vi "SubVI-Config-AI.vi"(8 "error in (no error)":errorcluster, 10 "Channels":T1(array[cluster])=[{" Physical Channel"="Dev2/ai0", "Name"="V_R", "Vmax"=10.0, "Vmin"=-10.0}, {" Physical Channel"="Dev2/ai1", "Name"="V_C", "Vmax"=10.0, "Vmin"=-10.0}, {" Physical Channel"="Dev2/ai2", "Name"="V_S", "Vmax"=10.0, "Vmin"=-10.0}], 11 "Timing Params":T2={"Trigger Level"=0.0, "Sample Rate"=0.0, "N Samples"=0, "Trigger Slope"=10280, "Enable"=FALSE} {"Trigger Slope" items=["Rising"=10171, "Falling"=10280]}) -> (0 "error out":errorcluster, 3 "Refnum out":refnum<k21>)   [LabVIEW 2023]
uses:
  <vilib>/DAQmx/create/channels.llb/DAQmx Create Channel (AI-Voltage-Basic).vi
  <vilib>/DAQmx/configure/timing.llb/DAQmx Timing (Sample Clock).vi
  <vilib>/DAQmx/configure/trigger.llb/DAQmx Start Trigger (Analog Edge).vi
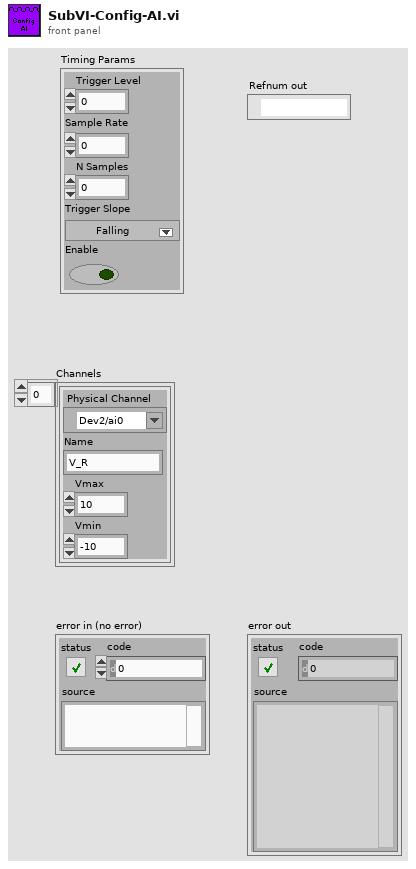
[diagram p1: front panel]
types:
  T1 = cluster{" Physical Channel":tag, "Name":string, "Vmax":dbl, "Vmin":dbl}[]
  T2 = cluster{"Trigger Level":dbl, "Sample Rate":dbl, "N Samples":i32, "Trigger Slope":i32, "Enable":bool}
  T3 = cluster{" Physical Channel":tag, "Name":string, "Vmax":dbl, "Vmin":dbl}
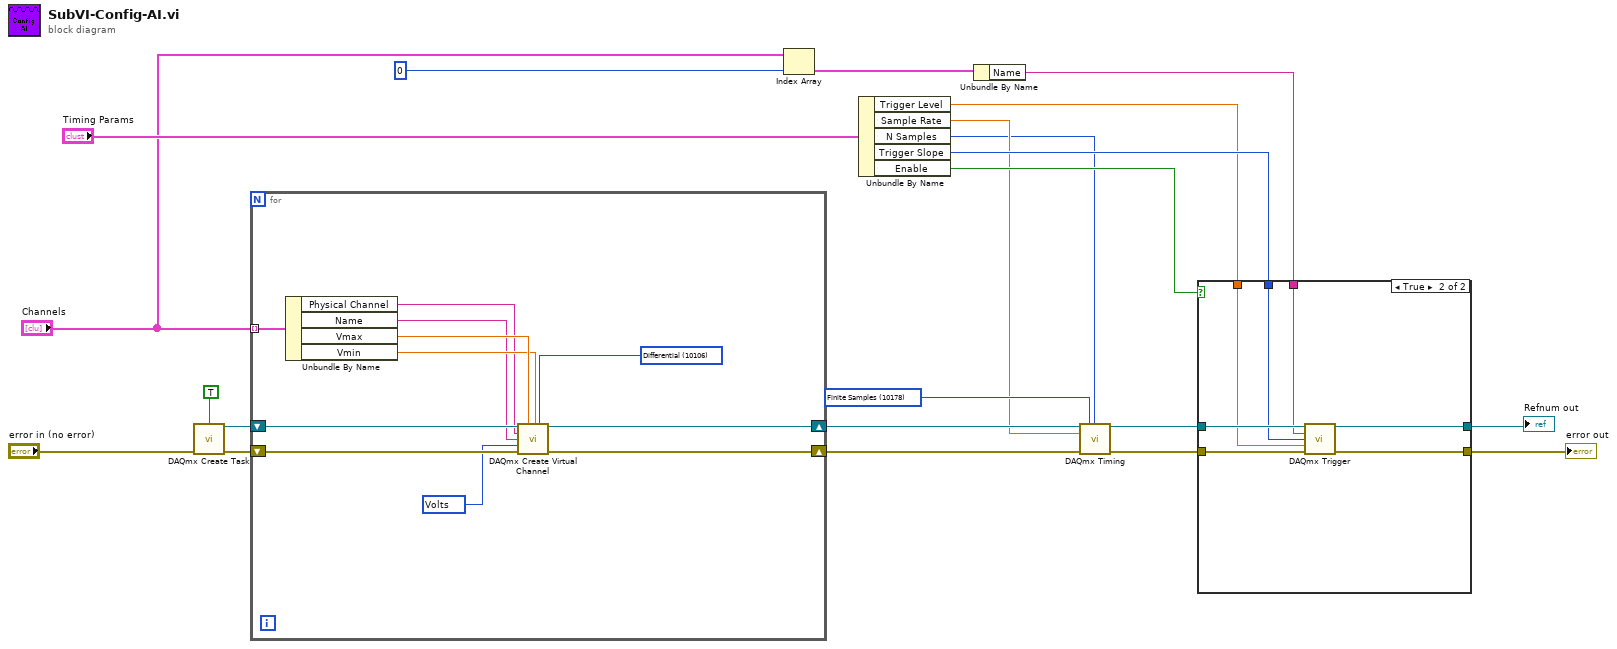
[diagram p0: block diagram]
diagram:
  w15 = 10178 items=["Finite Samples"=10178, "Continuous Samples"=10123, "Hardware Timed Single Point"=12522] ("sample mode")
  n1 = call <vilib>:"DAQmx Create Task.vi"("auto cleanup"=TRUE, "error in"="error in (no error)") -> ("task out"=w11:refnum<k21>, "error out"=w12:errorcluster)  [unwired: 12 in]
  n2 = for {
    tunnel: "Channels" -> [w29] mode=indexing
    shift-right: [w24] -> w14
    shift-left: w11 -> [w32]
    shift-right: [w23] -> w13
    shift-left: w12 -> [w31]
    w22 = 10348 items=["Volts"=10348, "From Custom Scale"=10065] ("units")
    w30 = 10106 items=["Default"=-1, "RSE"=10083, "NRSE"=10078, "Differential"=10106, "Pseudodifferential"=12529] ("input terminal configuration")
    n3 = Unbundle By Name(w29) -> ("Physical Channel"=w26:tag, "Name"=w25:string, "Vmax"=w28:dbl, "Vmin"=w27:dbl)
    n4 = call-poly <vilib>:"DAQmx Create Virtual Channel.vi"("task in"=w32, "maximum value"=w28, "minimum value"=w27, "input terminal configuration"=w30, "physical channels"=w26, "name to assign"=w25, "units"=w22, "error in"=w31) -> ("task out"=w24:refnum<k21>, "error out"=w23:errorcluster)  [unwired: 6 in]
  }
  n5 = Index Array(array="Channels", index=0) -> (element=w7:T3)
  n6 = Unbundle By Name("Timing Params") -> ("Trigger Level"=w4:dbl, "Sample Rate"=w2:dbl, "N Samples"=w1:i32, "Trigger Slope"=w9:i32, "Enable"=w3:bool)
  n7 = Unbundle By Name(w7) -> ("Name"=w6:string)
  n8 = call-poly <vilib>:"DAQmx Timing.vi"("task/channels in"=w14, "sample mode"=w15, "samples per channel"=w1, "rate"=w2, "error in"=w13) -> ("task out"=w17:refnum<k21>, "error out"=w19:errorcluster)  [unwired: 9 in]
  n9 = case shown="True" w3 {
    tunnel: w17 -> [w34 w41]
    tunnel: w19 -> [w33 w40]
    tunnel: [w34 w39] -> w20
    tunnel: [w33 w38] -> w21
    tunnel: w9 -> [_ w37]
    tunnel: w6 -> [_ w36]
    tunnel: w4 -> [_ w35]
    frame False {
    }
    frame True {
      n10 = call-poly <vilib>:"DAQmx Trigger.vi"("task/channels in"=w41, "source"=w36, "slope"=w37, "level"=w35, "error in"=w40) -> ("task out"=w39:refnum<k21>, "error out"=w38:errorcluster)  [unwired: 9 in]
    }
  }
  "error out" <- w21
  "Refnum out" <- w20
